vi "Analog Range.vi"(10 "ranges in":T1[](array[typedef])) -> (2 "range Array out":dbl[](array[numeric]))   [LabVIEW 2009, in "MicroDAQ.lvlib"]
uses:
  <instrlib>/MicroDAQ/MicroDAQ.lvlib
  <instrlib>/MicroDAQ/Tools/Analo Range Enum.ctl
panel:
  in  "ragne lookup table":dbl[][](array[numeric])=[[-10.0, 0.0, -5.0, 0.0, -5.12, -2.56, -2.5, -2.0, -1.24, -0.64], [10.0, 10.0, 5.0, 5.0, 5.12, 2.56, 2.5, 2.0, 1.24, 0.64]]
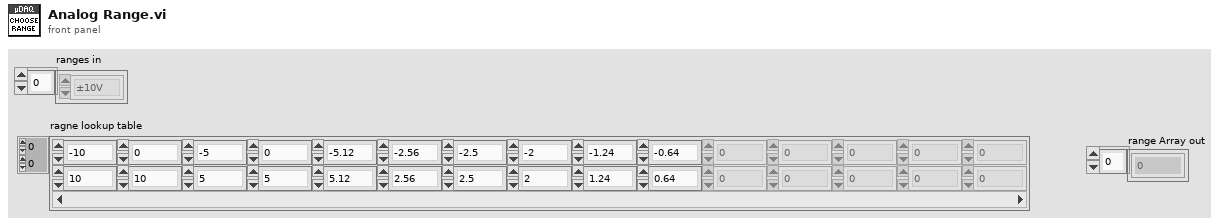
[diagram p1: front panel]
types:
  T1 = typedef "MicroDAQ.lvlib/Analo Range Enum.ctl" = enum16{"±10V", "0-10V", "±5V", "0-5V", "±5.12V", "±2.56V", "±2.5V", "±2V", "±1.24V", "±0.64V"}
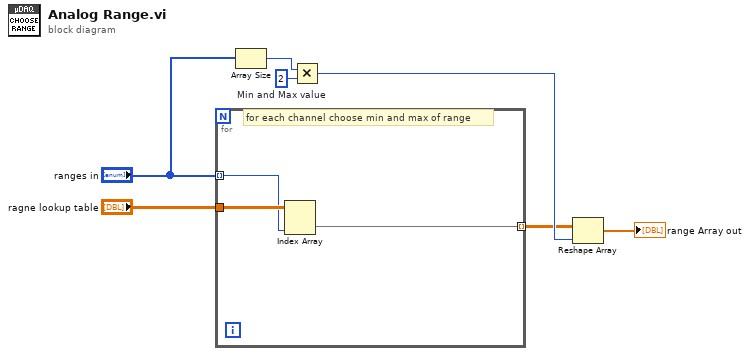
[diagram p0: block diagram]
diagram:
  w7 = 2  # Min and Max value
  n1 = for {
    tunnel: "ragne lookup table" -> [w10]
    tunnel: "ranges in" -> [w9] mode=indexing
    tunnel: [w8] -> w2 mode=indexing
    # "for each channel choose min and max of range"
    n2 = Index Array(array=w10, index (col)=w9) -> (element=w8:dbl[])  [unwired: 1 in]
  }
  n3 = Array Size(array="ranges in") -> (size(s)=w3:i32)
  n4 = Multiply(x=w3, y=w7) -> (x*y=w6:i32)
  n5 = Reshape Array(w2, w6) -> (→"range Array out":dbl[])
